vi "Acquire_wpulser.vi"(0 "Ch Armed Reg":refnum<k21>="Register 1", 1 "Command FIFO":refnum<k21>="To DMA FIFO", 3 "Circular Buffer Mem":refnum<k21>, 4 "circular buffer length":u32=300, 5 "FPGA I/O In":refnum<k21>="IO Module\\AI A0", 6 "with dead time":bool=TRUE, 7 "channel on/off":bool, 9 "Trigger":i16=1500, 10 "Timing FIFO":refnum<k21>, 11 "Records to Acquire":u32=100, 12 "Simulate":bool, 13 "Is test pulse?":bool, 14 "# of pretrigger":u32=15, 15 "timing":u64) -> (8 "Is digitizing?":bool)   [LabVIEW 2012]
uses:
  <vilib>/rvi/DataTransferAndStorage/Container/Common/niFpgaContainerExecOnDevCompGetState.vi
  <vilib>/rvi/Memory/Memory_Emulation/nirvimemoryEmulationManagerCache_GetValue.vi
  <vilib>/rvi/Memory/Memory_Emulation/niFpgaMemoryEmulationValidateCache.vi
  <vilib>/rvi/DataTransferAndStorage/Container/Common/niFpgaContainerGetUniqueNameForEmu.vi
  <vilib>/rvi/Memory/Memory_Emulation/nirvimemoryEmulationManagerCache_InsertValue.vi
  <vilib>/rvi/eio/common/nirviEmuTemplateMethod_errors.vi
  <vilib>/rvi/Emulation/niFpgaSctlEmulationGetInTimedLoop.vi
  <vilib>/rvi/FIFO/Fifo_Resource/nirvififoEmulationSetSize.vi
  <vilib>/rvi/errors/niFpgaSetErrorForExecOnDevCompSimple.vi
  <vilib>/rvi/eio/common/nirviEmuReportErrorAndStop.vi
  <vilib>/rvi/Emulation/niFpgaSctlEmulationFifoFullMgr.vi
  <vilib>/rvi/Emulation/niFpgaSctlEmulationResourceMgr.vi
  <vilib>/rvi/interface/RandomDataEmulation/nirviRandomDataFPGAFIFO.vi
  <vilib>/rvi/interface/RandomDataEmulation/niFpgaRandomDataHandleErrors.vi
  <vilib>/rvi/DataTransferAndStorage/Container/XNode/niFpgaContainer.xnode
  <vilib>/rvi/DataTransferAndStorage/Register/Emulation/niFpgaRegisterEmulationRefIn.vi
  <vilib>/eio/EIONode/EIONode.xnode
  <vilib>/rvi/FIFO/Fifo_Resource/niFpgaFifoEmulationRefIn.vi
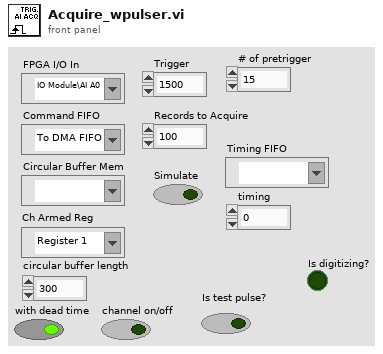
[diagram p1: front panel]
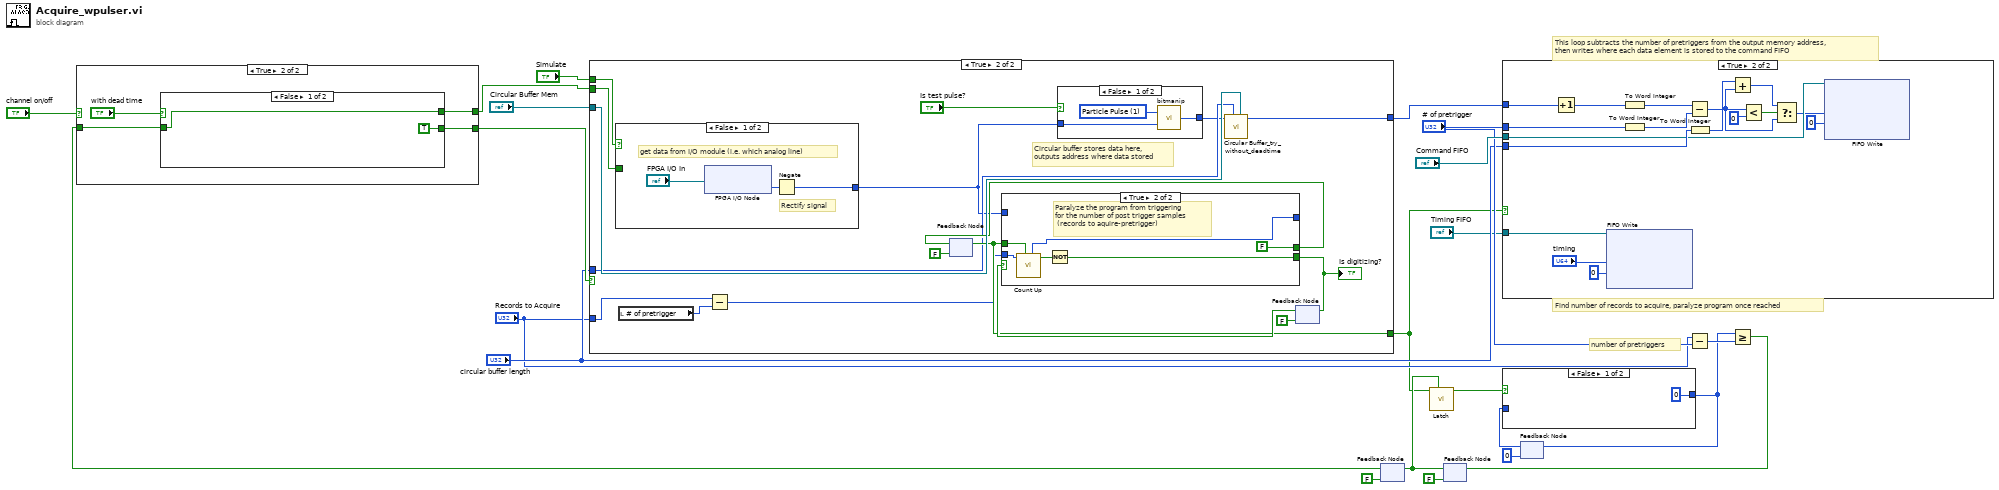
[diagram p0: block diagram]
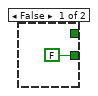
[diagram p2: hidden frame]
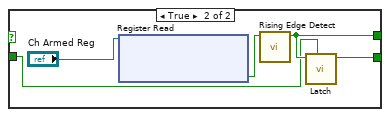
[diagram p3: hidden frame]
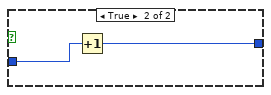
[diagram p4: hidden frame]
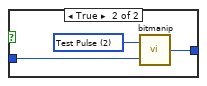
[diagram p6: hidden frame]
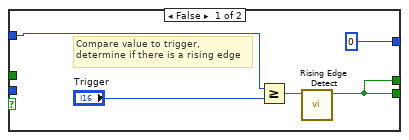
[diagram p7: hidden frame]
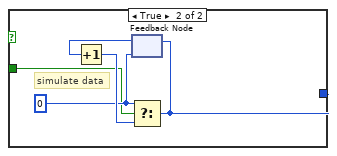
[diagram p8: hidden frame]
diagram:
  # "This loop subtracts the number of pretriggers from the output memory address, \nthen writes where each data element is stored to the command FIFO"
  # "Find number of records to acquire, paralyze program once reached"
  # "number of pretriggers"
  n1 = feedback #1(FALSE ("Count Met")) -> (w12:bool)
  n2 = case shown="True" "channel on/off" {
    tunnel: [FALSE ("Output") w27] -> w19
    tunnel: [_ w26] -> w18
    tunnel: w12 -> [_ w25]
    frame False {
    }
    frame True {
      n3 = case shown="False" "with dead time" {
        tunnel: [TRUE ("Output") w33] -> w27
        tunnel: [w29 w31] -> w26
        tunnel: w25 -> [w29 w30]
        frame False {
        }
        frame True {
          n4 = xnode ("Register Read")("Register In"="Ch Armed Reg") -> ("Data"=w32:bool)  [unwired: 1 out]
          n5 = call "Rising Edge Detect.vi"("Input"=w32) -> ("Rising Edge"=w31:bool)  [unwired: 10 in]
          n6 = call "Latch.vi"("Reset"=w30, "Input"=w31) -> ("Output"=w33:bool)  [unwired: 9 in]
        }
      }
    }
  }
  n7 = case shown="True" w19 {
    tunnel: "Circular Buffer Mem" -> [_ w51]
    tunnel: "circular buffer length" -> [_ w41]
    tunnel: [_ w50] -> w20
    tunnel: w18 -> [_ w49]
    tunnel: "Simulate" -> [_ w48]
    tunnel: "Records to Acquire" -> [_ w37]
    tunnel: [_ w43] -> w1
    frame False {
    }
    frame True {
      # "Circular buffer stores data here, \noutputs address where data stored"
      n8 = case shown="False" w48 {
        tunnel: [w69 w73] -> w40
        tunnel: w49 -> [_ w72]
        frame False {
          # "Rectify signal"
          # "get data from I/O module (i.e. which analog line)"
          n9 = xnode "FPGA I/O Node"("FPGA I/O In"="FPGA I/O In") -> ("I/O Item"=w71:i16)  [unwired: 1 out]
          n10 = Negate(x=w71) -> (-x=w69:i16)
        }
        frame True {
          w74 = i16 0 ("x")
          # "simulate data"
          n11 = feedback #2(w74) -> (w76:i16)
          n12 = Increment(x=w76) -> (x+1=w75:i16)
          n13 = Select(t=w74, s=w72, f=w75) -> (s? t:f=w73:i16)
          n14 = feedback-in #2(w73) -> ()
        }
      }
      n15 = local read "# of pretrigger"() -> (w35:u32)
      n16 = Subtract(x=w37, y=w35) -> (x-y=w36:u32)
      n17 = feedback #3(FALSE ("Rising Edge")) -> (w43:bool)
      n18 = case shown="False" "Is test pulse?" {
        tunnel: w40 -> [w53 w56]
        tunnel: [w54 w55] -> w39
        frame False {
          w52 = u16 1 items=["Header Information", "Particle Pulse", "Test Pulse"] ("Pulse Type")
          n19 = call "bitmanip.vi"("Pulse Type"=w52, "Integer to be written"=w53) -> ("Integer Written"=w54:i16)  [unwired: 2 in]
        }
        frame True {
          w57 = u16 2 items=["Header Information", "Particle Pulse", "Test Pulse"] ("Pulse Type")
          n20 = call "bitmanip.vi"("Pulse Type"=w57, "Integer to be written"=w56) -> ("Integer Written"=w55:i16)  [unwired: 2 in]
        }
      }
      n21 = call "Circular Buffer_try_without_deadtime.vi"("Refnum in"=w51, "circular buffer length"=w41, "Data"=w39) -> ("Address"=w50:u16)  [unwired: 8 in]
      n22 = feedback #4(FALSE ("Rising Edge")) -> (w47:bool)
      n23 = case shown="True" w47 {
        tunnel: w40 -> [w62 _]
        tunnel: [w59 w66] -> w45
        tunnel: w36 -> [_ w68]
        tunnel: [w59 FALSE ("Rising Edge")] -> w44
        tunnel: w43 -> [_ w65]
        tunnel: [u32 0 ("count") w63] -> _
        frame False {
          # "Compare value to trigger, \ndetermine if there is a rising edge"
          n24 = Greater Or Equal?(x=w62, y="Trigger") -> (x >= y?=w60:bool)
          n25 = call "Rising Edge Detect.vi"("Input"=w60) -> ("Rising Edge"=w59:bool)  [unwired: 10 in]
        }
        frame True {
          # "Paralyze the program from triggering \nfor the number of post trigger samples\n (records to aquire-pretrigger)"
          n26 = call "Count Up.vi"("Reset?"=w65, "goal"=w68) -> ("Count Met"=w67:bool, "count"=w63:u32)  [unwired: 8 in]
          n27 = Not(x=w67) -> (.not. x?=w66:bool)
        }
      }
      "Is digitizing?" <- w45
      n28 = feedback-in #3(w44) -> ()
      n29 = feedback-in #4(w45) -> ()
    }
  }
  n30 = feedback #5(FALSE) -> (w14:bool)
  n31 = feedback-in #1(w14) -> ()
  n32 = call "Latch.vi"("Reset"=w14, "Input"=w1) -> ("Output"=w11:bool)  [unwired: 9 in]
  n33 = case shown="True" w1 {
    tunnel: "Command FIFO" -> [_ w78]
    tunnel: w20 -> [_ w81]
    tunnel: "# of pretrigger" -> [_ w82]
    tunnel: "circular buffer length" -> [_ w80]
    tunnel: "Timing FIFO" -> [_ w93]
    frame False {
    }
    frame True {
      n34 = Increment(x=w81) -> (x+1=w88:u16)
      n35 = xnode ("FIFO Write")("Element"="timing", "Timeout"=0, "FIFO In"=w93) -> ()  [unwired: 2 out]
      n36 = To Word Integer(number=w88) -> (16bit integer=w89:i16)
      n37 = To Word Integer(number=w82) -> (16bit integer=w90:i16)
      n38 = Subtract(x=w89, y=w90) -> (x-y=w86:i16)
      n39 = To Word Integer(number=w80) -> (16bit integer=w87:i16)
      n40 = Add(x=w87, y=w86) -> (x+y=w85:i16)
      n41 = Less?(x=w86, y=i16 0) -> (x < y?=w83:bool)
      n42 = Select(t=w85, s=w83, f=w86) -> (s? t:f=w77:i16)
      n43 = xnode ("FIFO Write")("Element"=w77, "Timeout"=0, "FIFO In"=w78) -> ()  [unwired: 2 out]
    }
  }
  n44 = feedback #6(u32 0) -> (w7:u32)
  n45 = case shown="False" w11 {
    tunnel: [u32 0 w96] -> w5
    tunnel: w7 -> [_ w95]
    frame False {
    }
    frame True {
      n46 = Increment(x=w95) -> (x+1=w96:u32)
    }
  }
  n47 = feedback-in #6(w5) -> ()
  n48 = Subtract(x="Records to Acquire", y="# of pretrigger") -> (x-y=w10:u32)
  n49 = Greater Or Equal?(x=w5, y=w10) -> (x >= y?=w9:bool)
  n50 = feedback-in #5(w9) -> ()
